vi "Tektronix DPO MSO 2000 4000 Series Acquire Continuous Waveform Example.vi"() -> ()   [LabVIEW 2010]
doc: "This example illustrates how to use autosetup and continuously acquires waveforms from a single channel using the following steps:\n\n1. Specify a valid VISA session. \n2. Specify a channel. \n3. Specify a time-out value for reading waveform.\n4. Run the VI. The graph displays the waveform you acquire."
uses:
  <instrlib>/Tektronix DPO MSO 2000 4000 Series/Public/Data/Read (Single Waveform).vi
  <instrlib>/Tektronix DPO MSO 2000 4000 Series/Tektronix DPO MSO 2000 4000 Series.lvlib
panel:
  in  "Channel (0: Channel 1)":u16(ring) items=["Channel 1", "Channel 2", "Channel 3", "Channel 4", "Math", "Reference 1", "Reference 2", "Reference 3", "Reference 4"]
  in  "Maximum Time (10000ms)":u32=10000
  in  "stop":bool
  in  "VISA Resource Name":refnum<visa-resource-name>
  out "Waveform Graph":waveform(dbl)(graph)
  # "(c) 2006 - 2012. National Instruments Corporation. ALL RIGHTS RESERVED."
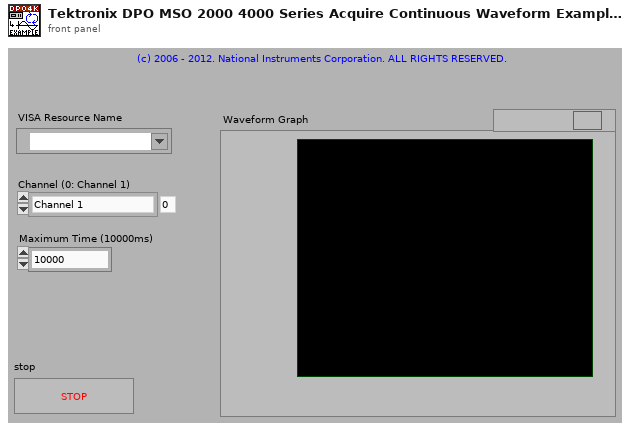
[diagram p1: front panel]
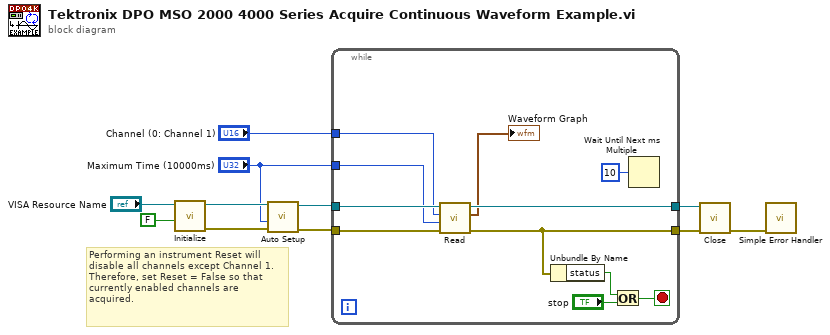
[diagram p0: block diagram]
diagram:
  # "Performing an instrument Reset will disable all channels except Channel 1. Therefore, set Reset = False so that currently enabled channels are acquired."
  n1 = call <instrlib>:"Initialize.vi"("Reset (True)"=FALSE, "VISA resource name"="VISA Resource Name") -> ("error out"=w4:errorcluster, "VISA resource name out"=w5:refnum<visa-resource-name>)  [unwired: 8 in]
  n2 = call <instrlib>:"Auto Setup.vi"("error in (no error)"=w4, "Maximum Time (10000ms)"="Maximum Time (10000ms)", "VISA resource name"=w5) -> ("error out"=w6:errorcluster, "VISA resource name out"=w7:refnum<visa-resource-name>)  [unwired: 7 in]
  n3 = while {
    tunnel: w7 -> [w22]
    tunnel: w6 -> [w21]
    tunnel: [w20] -> w10
    tunnel: [w18] -> w9
    tunnel: "Maximum Time (10000ms)" -> [w14]
    tunnel: "Channel (0: Channel 1)" -> [w12]
    stop <- w15 stop-if-true
    n4 = call-poly <instrlib>:"Read.vi"("error in (no error)"=w21, "Maximum Time (10000ms)"=w14, "Channel (0: Channel 1)"=w12, "VISA resource name"=w22) -> ("error out"=w18:errorcluster, "Waveform Graph"=→"Waveform Graph":waveform(dbl), "VISA resource name out"=w20:refnum<visa-resource-name>)  [unwired: 5 in]
    n5 = Unbundle By Name(w18) -> ("status"=w17:bool)
    n6 = Or(x=w17, y="stop") -> (x .or. y?=w15:bool)
    n7 = Wait Until Next ms Multiple(millisecond multiple=u32 10) -> ()  [unwired: 1 out]
  }
  n8 = call <instrlib>:"Close.vi"("error in (no error)"=w9, "VISA resource name"=w10) -> ("error out"=w8:errorcluster)  [unwired: 9 in]
  n9 = call <vilib>:"Simple Error Handler.vi"("error in (no error)"=w8) -> ()  [unwired: 4 in, 5 out]
